vi "Low Sampling to the Extreme.vi"() -> ()   [LabVIEW 2025]
uses:
  <vilib>/Analysis/2dsp.llb/Real FFT.vi
  <vilib>/Analysis/NI_AALBase.lvlib
  <vilib>/Analysis/NI_AALPro.lvlib
panel:
  out "The Spectrum 2":dbl[](graph)
  out "The Spectrum":dbl[](graph)
  out "The Signal":cluster{"Sinusoidal Pattern":dbl[]}[](graph)
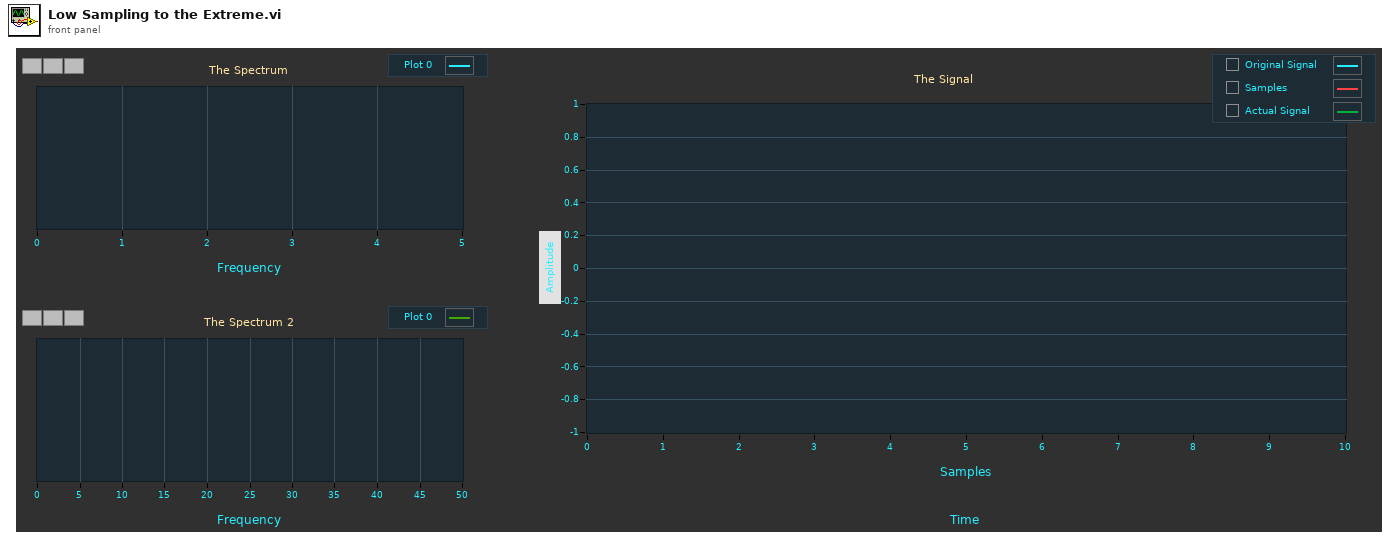
[diagram p1: front panel]
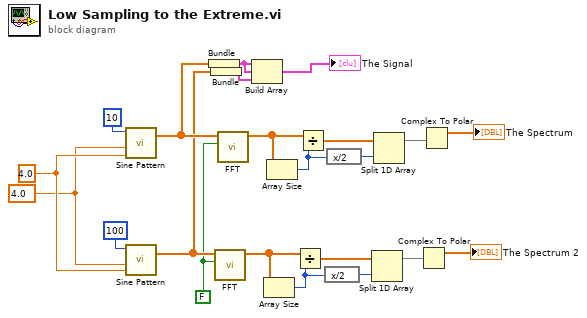
[diagram p0: block diagram]
diagram:
  w16 = 4.0 ("cycles")
  w12 = 4.0 ("phase(degrees)")
  w8 = FALSE ("shift?")
  n1 = call <vilib>:"Sine Pattern.vi"("cycles"=w16, "phase(degrees)"=w12, "samples"=10) -> ("Sinusoidal Pattern"=w21:dbl[])  [unwired: 1 in, 1 out]
  n2 = call <vilib>:"Sine Pattern.vi"("cycles"=w16, "phase(degrees)"=w12, "samples"=100) -> ("Sinusoidal Pattern"=w13:dbl[])  [unwired: 1 in, 1 out]
  n3 = Bundle("Sinusoidal Pattern"=w21) -> (w1:cluster{"Sinusoidal Pattern":dbl[]})  [unwired: 1 in]
  n4 = Bundle("Sinusoidal Pattern"=w13) -> (w2:cluster{"Sinusoidal Pattern":dbl[]})  [unwired: 1 in]
  n5 = call-poly <vilib>:"FFT.vi"("shift?"=w8, "X"=w13) -> ("FFT {X}"=w18:cdb[])  [unwired: 8 in, 1 out]
  n6 = call-poly <vilib>:"FFT.vi"("shift?"=w8, "X"=w21) -> ("FFT {X}"=w22:cdb[])  [unwired: 8 in, 1 out]
  n7 = Build Array(w1, w1, w2) -> (→"The Signal":cluster{"Sinusoidal Pattern":dbl[]}[])
  n8 = Array Size(array=w18) -> (size(s)=w3:i32)
  n9 = Array Size(array=w22) -> (size(s)=w4:i32)
  n10 = Divide(x=w18, y=w3) -> (x/y=w10:cdb[])
  n11 = Divide(x=w22, y=w4) -> (x/y=w9:cdb[])
  n12 = expression code="x/2"(w3) -> (w11:i32)
  n13 = expression code="x/2"(w4) -> (w5:i32)
  n14 = Split 1D Array(array=w10, index=w11) -> (first subarray=w7:cdb[])  [unwired: 1 out]
  n15 = Split 1D Array(array=w9, index=w5) -> (first subarray=w6:cdb[])  [unwired: 1 out]
  n16 = Complex To Polar(r * e^(i*theta)=w7) -> (r=→"The Spectrum 2":dbl[])  [unwired: 1 out]
  n17 = Complex To Polar(r * e^(i*theta)=w6) -> (r=→"The Spectrum":dbl[])  [unwired: 1 out]
